vi "Broadcast FG.vi"(7 "Broadcast Actions":T2=enum."Get", 8 "error in":errorcluster) -> (0 "error out":errorcluster, 3 "Broadcast List":T1)   [LabVIEW 2015, in "Generic Module Library.lvlib" / "Template G_Module.lvlib"]
uses:
  Template G_Module.lvlib
  Private Controls/Event Item.ctl
  API/Broadcast List.ctl
  Broadcast Actions.ctl
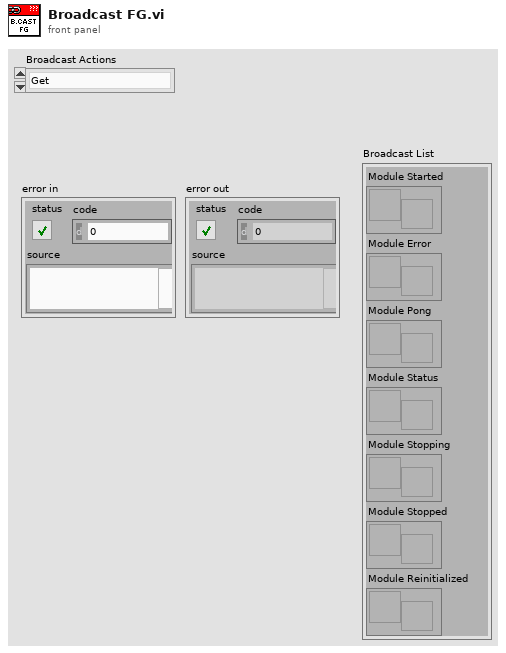
[diagram p1: front panel]
types:
  T1 = typedef "Generic Module Library.lvlib/Template G_Module.lvlib/Broadcast List.ctl" = cluster{"Module Started":refnum<user-event>, "Module Error":refnum<user-event>, "Module Pong":refnum<user-event>, "Module Status":refnum<user-event>, "Module Stopping":refnum<user-event>, "Module Stopped":refnum<user-event>, "Module Reinitialized":refnum<user-event>}
  T2 = typedef "Generic Module Library.lvlib/Template G_Module.lvlib/Broadcast Actions.ctl" = enum16{"Create", "Get", "Destroy"}
  T3 = typedef "Generic Module Library.lvlib/Template G_Module.lvlib/Event Item.ctl" = cluster{"Event Data":variant}
  T4 = cluster{"[0]":refnum<user-event>, "[1]":refnum<user-event>, "[2]":refnum<user-event>, "[3]":refnum<user-event>, "[4]":refnum<user-event>, "[5]":refnum<user-event>, "[6]":refnum<user-event>, "[7]":refnum<user-event>, "[8]":refnum<user-event>}
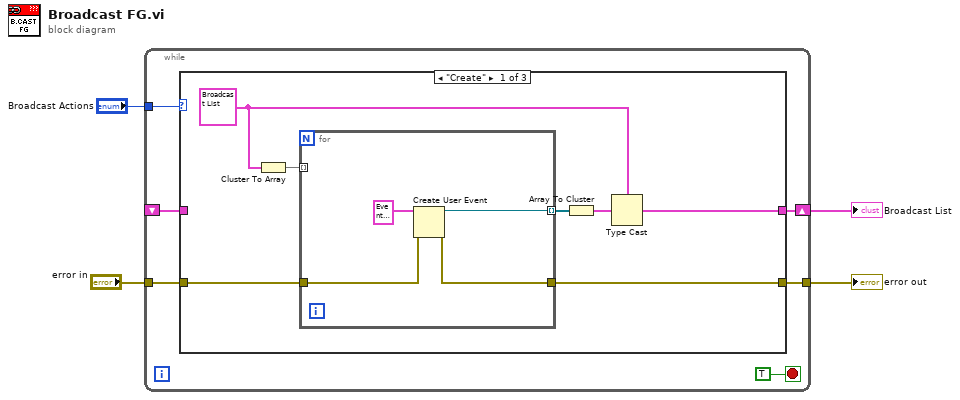
[diagram p0: block diagram]
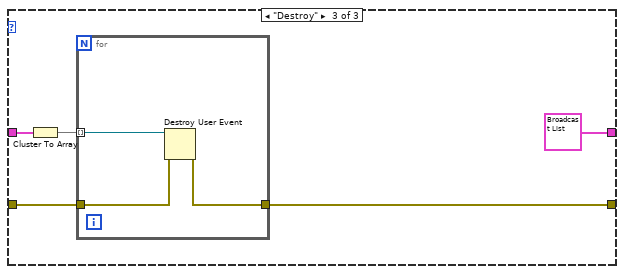
[diagram p3: hidden frame]
diagram:
  n1 = while {
    tunnel: "Broadcast Actions" -> [w9]
    tunnel: "error in" -> [w8]
    tunnel: [w7] -> w3
    shift-right: [w6] -> w1
    shift-left: _ -> [w5]
    stop <- TRUE stop-if-true
    n2 = case shown="\"Create\"" w9 {
      tunnel: w8 -> [w17 w23 w28]
      tunnel: [w16 w23 w27] -> w7
      tunnel: [w11 w22 T1 {"Module Started"=refnum, "Module Error"=refnum, "Module Pong"=refnum, "Module Status"=refnum, "Module Stopping"=refnum, "Module Stopped"=refnum, "Module Reinitialized"=refnum} ("Broadcast List")] -> w6
      tunnel: w5 -> [_ w22 w26]
      frame "Create" {
        w12 = T1 {"Module Started"=refnum, "Module Error"=refnum, "Module Pong"=refnum, "Module Status"=refnum, "Module Stopping"=refnum, "Module Stopped"=refnum, "Module Reinitialized"=refnum} ("Broadcast List")
        n3 = Cluster To Array(cluster=w12) -> (array=w15:refnum<user-event>[])
        n4 = for {
          tunnel: [w21] -> w16
          tunnel: w17 -> [w20]
          tunnel: [w18] -> w14 mode=indexing
          tunnel: w15 -> [_] mode=indexing
          n5 = Create User Event(user event datatype=T3 {"Event Data"=variant} ("Broadcast Item"), error in=w20) -> (user event=w18:refnum<user-event>, error out=w21:errorcluster)
        }
        n6 = Array To Cluster(array=w14) -> (cluster=w13:T4)
        n7 = Type Cast(type=w12, x=w13) -> (*(type *) &x=w11:T1)
      }
      frame "Get", Default {
      }
      frame "Destroy" {
        n8 = Cluster To Array(cluster=w26) -> (array=w25:refnum<user-event>[])
        n9 = for {
          tunnel: [w31] -> w27
          tunnel: w28 -> [w29]
          tunnel: w25 -> [w30] mode=indexing
          n10 = Destroy User Event(user event=w30, error in=w29) -> (error out=w31:errorcluster)
        }
      }
    }
  }
  "error out" <- w3
  "Broadcast List" <- w1
